vi "Get FIFO Offsets by Name and DataType.vi"(6 "offset":i32, 7 "User Specified?":bool, 8 "error in":errorcluster, 9 "HostToTarget FIFOs":string[](array[string]), 10 "TargetToHost FIFOs":string[](array[string]), 11 "bitfile xml in":string) -> (0 "error out":errorcluster, 1 "HostToTarget":T2, 2 "TargetToHost":T2, 4 "offset past EndTag":i32, 5 "All FIFOs":T1[](array[typedef]))   [LabVIEW 2010, in "FPGA Bitfile Utility.lvlib"]
uses:
  <userlib>/_FPGA Interface Advanced Tools/FPGA Bitfile Utility/FPGA Bitfile Utility.lvlib
  <userlib>/_FPGA Interface Advanced Tools/FPGA Bitfile Utility/TypeDefs/FIFO Channel Set.ctl
  <userlib>/_FPGA Interface Advanced Tools/FPGA Bitfile Utility/TypeDefs/FIFO Channel.ctl
  <vilib>/rvi/DataTransferAndStorage/Container/Common/niFpgaDataTypeControl.ctl
  <userlib>/_FPGA Interface Advanced Tools/FPGA Bitfile Utility/Get FIFOs.vi
  <vilib>/rvi/Utilities/XML/nirviXML_GetValue.vi
  <vilib>/rvi/Utilities/XML/nirviXML_GetValue_String.vi
  resource/RVI/compilationResultUtilities/niLvFpgaGetDmaChannelInfoFromXML.vi
  <vilib>/Utility/error.llb/Error Cluster From Error Code.vi
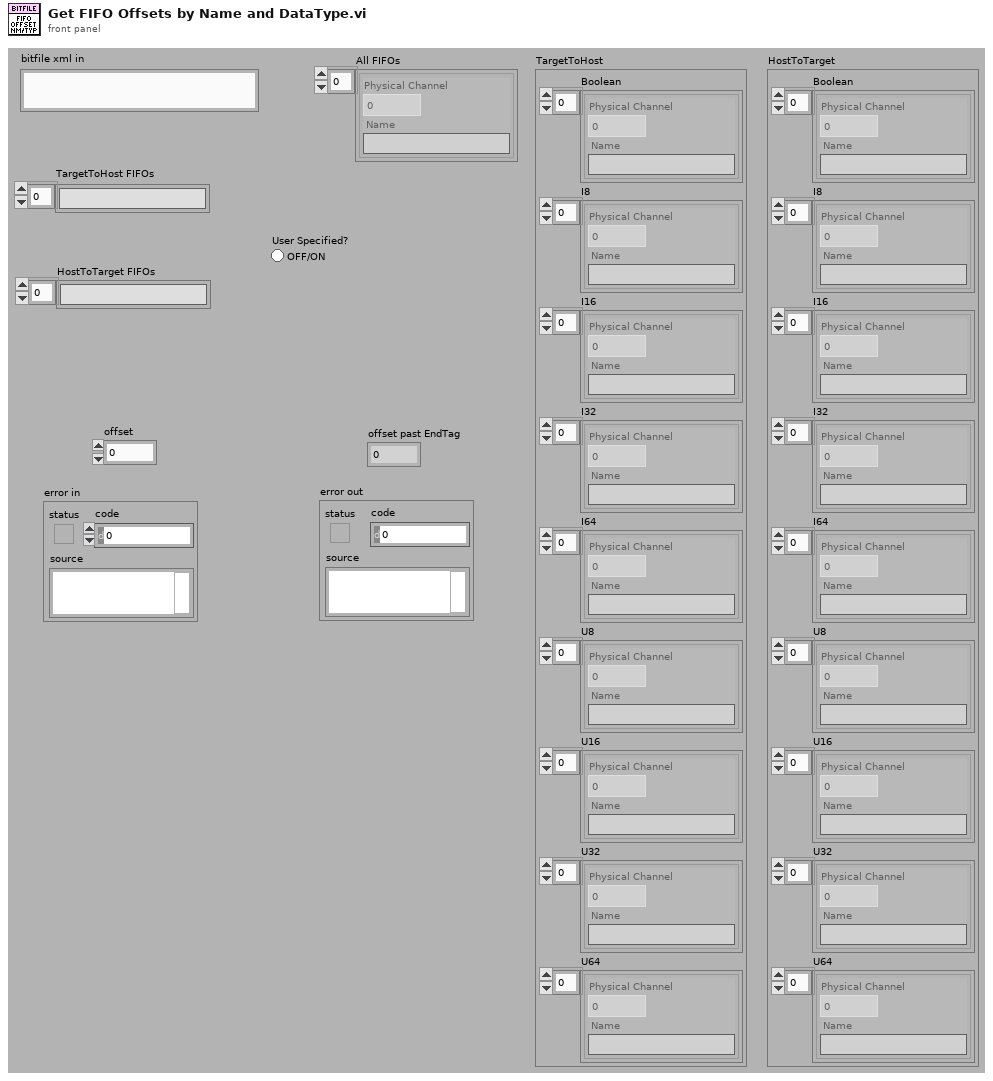
[diagram p1: front panel]
types:
  T1 = typedef "FPGA Bitfile Utility.lvlib/FIFO Channel.ctl" = cluster{"Physical Channel":u32, "Name":string}
  T2 = typedef "FPGA Bitfile Utility.lvlib/FIFO Channel Set.ctl" = cluster{"Boolean":T1[], "I8":T1[], "I16":T1[], "I32":T1[], "I64":T1[], "U8":T1[], "U16":T1[], "U32":T1[], "U64":T1[]}
  T3 = typedef "FPGA Bitfile Utility.lvlib/FIFO Info.ctl" = cluster{"Data Type":T4, "Physical Channel":u32, "Name":string}
  T4 = typedef "niFpgaDataTypeControl.ctl" = enum32{"Boolean", "I8", "I16", "I32", "I64", "U8", "U16", "U32", "U64", "FXP", "CustomControl"}
  T5 = cluster{T1[], T1[], T1[], T1[], T1[], T1[], T1[], T1[], T1[]}
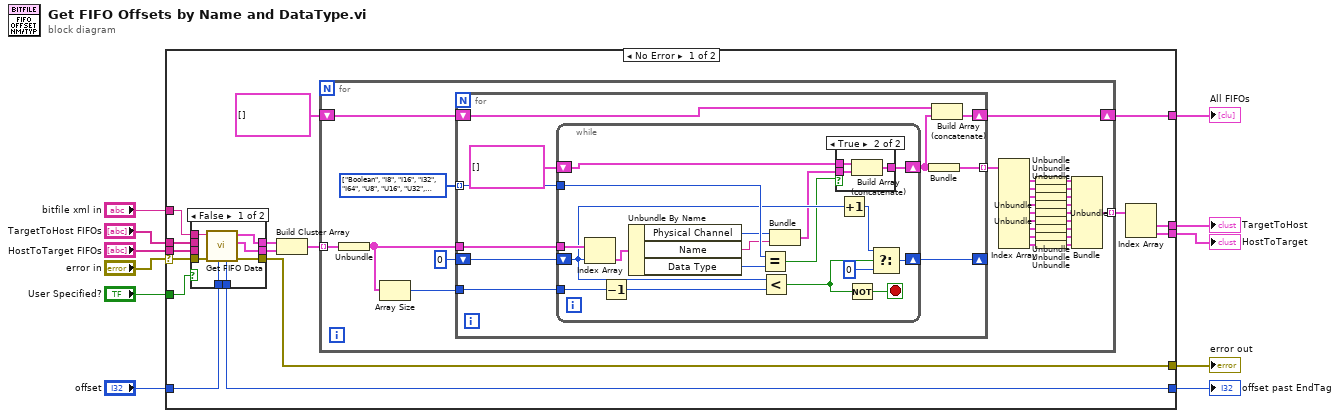
[diagram p0: block diagram]
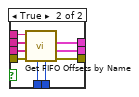
[diagram p2: hidden frame]
diagram:
  n1 = case shown="No Error" "error in" {
    selector: "error in" -> [w20 w104]
    tunnel: [w25 _] -> w4
    tunnel: [w24 _] -> w3
    tunnel: [w21 w104] -> w10
    tunnel: "bitfile xml in" -> [w15 _]
    tunnel: "TargetToHost FIFOs" -> [w19 _]
    tunnel: "HostToTarget FIFOs" -> [w18 _]
    tunnel: "offset" -> [w17 w103]
    tunnel: [w16 w103] -> w5
    tunnel: [w13 _] -> w2
    tunnel: "User Specified?" -> [w12 _]
    frame No Error {
      n2 = case shown="False" w12 {
        tunnel: [w30 w43] -> w23
        tunnel: [w29 w42] -> w22
        tunnel: [w28 w41] -> w21
        tunnel: w20 -> [w31 w40]
        tunnel: w19 -> [_ w39]
        tunnel: w18 -> [_ w38]
        tunnel: w17 -> [w33 w37]
        tunnel: [w32 w36] -> w16
        tunnel: w15 -> [w34 w35]
        frame False {
          n3 = call <userlib>:"Get FIFO Data.vi"("offset"=w33, "error in (no error)"=w31, "bitfile xml in"=w34) -> ("error out"=w28:errorcluster, "HostToTargetFIFOs"=w29:T3[], "TargetToHost FIFOs"=w30:T3[], "offset past EndTag"=w32:i32)  [unwired: 5 in]
        }
        frame True {
          n4 = call <userlib>:"Get FIFO Offsets by Name.vi"("offset"=w37, "error in (no error)"=w40, "HostToTarget FIFOs"=w38, "TargetToHost FIFOs"=w39, "bitfile xml in"=w35) -> ("error out"=w41:errorcluster, "HostToTarget FIFO Offsets"=w42:T3[], "TargetToHost FIFO Offsets"=w43:T3[], "offset past EndTag"=w36:i32)  [unwired: 3 in]
        }
      }
      n5 = Build Cluster Array(w23, w22) -> (w27:cluster{"HostToTarget FIFO Offsets":T3[]}[])
      n6 = for {
        tunnel: w27 -> [w70] mode=indexing
        tunnel: [w46] -> w26 mode=indexing
        shift-right: [w45] -> w13
        shift-left: T1[] [] -> [w44]
        w69 = T4[] [enum."Boolean", enum."I8", enum."I16", enum."I32", enum."I64", enum."U8", enum."U16", enum."U32", enum."U64"] items=["Boolean", "I8", "I16", "I32", "I64", "U8", "U16", "U32", "U64", "FXP", "CustomControl"]
        n7 = Unbundle(w70) -> ("HostToTarget FIFO Offsets"=w66:T3[])
        n8 = Array Size(array=w66) -> (size(s)=w67:i32)
        n9 = for {
          tunnel: w69 -> [w80] mode=indexing
          tunnel: w66 -> [w79]
          shift-right: [w77] -> _
          shift-left: 0 -> [w78]
          tunnel: [w76] -> w47 mode=indexing
          tunnel: w67 -> [w74]
          shift-right: [w72] -> w45
          shift-left: w44 -> [w71]
          n10 = while {
            tunnel: w80 -> [w94]
            tunnel: w79 -> [w98]
            shift-right: [w96] -> w77
            shift-left: w78 -> [w88]
            shift-right: [w92] -> w73
            shift-left: T1[] [] -> [w91]
            tunnel: w74 -> [w89]
            stop <- w90 stop-if-true
            n11 = Index Array(array=w98, index=w88) -> (element=w93:T3)
            n12 = Decrement(x=w89) -> (x-1=w84:i32)
            n13 = Unbundle By Name(w93) -> ("Physical Channel"=w87:u32, "Name"=w86:string, "Data Type"=w95:T4)
            n14 = Equal?(x=w94, y=w95) -> (x = y?=w82:bool)
            n15 = Less?(x=w88, y=w84) -> (x < y?=w83:bool)
            n16 = Bundle("Physical Channel"=w87, "Name"=w86) -> (w85:cluster{"Physical Channel":u32, "Name":string})  [unwired: 1 in]
            n17 = case shown="True" w82 {
              tunnel: w85 -> [_ w102]
              tunnel: [w99 w101] -> w92
              tunnel: w91 -> [w99 w100]
              frame False {
              }
              frame True {
                n18 = Build Array (concatenate)(w100, w102) -> (w101:T1[])
              }
            }
            n19 = Increment(x=w88) -> (x+1=w97:i32)
            n20 = Not(x=w83) -> (.not. x?=w90:bool)
            n21 = Select(t=w97, s=w83, f=0) -> (s? t:f=w96:i32)
          }
          n22 = Bundle(w73) -> (w76:cluster{T1[]})  [unwired: 1 in]
          n23 = Build Array (concatenate)(w71, w73) -> (w72:T1[])
        }
        n24 = Index Array(array=w47) -> (element #1=w48:cluster{T1[]}, element #2=w50:cluster{T1[]}, element #3=w52:cluster{T1[]}, element #4=w53:cluster{T1[]}, element #5=w56:cluster{T1[]}, element #6=w57:cluster{T1[]}, element #7=w58:cluster{T1[]}, element #8=w59:cluster{T1[]}, element #9=w60:cluster{T1[]})  [unwired: 9 in]
        n25 = Unbundle(w48) -> (w49:T1[])
        n26 = Unbundle(w50) -> (w51:T1[])
        n27 = Unbundle(w52) -> (w55:T1[])
        n28 = Unbundle(w53) -> (w54:T1[])
        n29 = Unbundle(w56) -> (w65:T1[])
        n30 = Unbundle(w57) -> (w64:T1[])
        n31 = Unbundle(w58) -> (w63:T1[])
        n32 = Unbundle(w59) -> (w62:T1[])
        n33 = Unbundle(w60) -> (w61:T1[])
        n34 = Bundle(w49, w51, w55, w54, w65, w64, w63, w62, w61) -> (w46:T5)  [unwired: 1 in]
      }
      n35 = Index Array(array=w26) -> (element #1=w25:T5, element #2=w24:T5)  [unwired: 2 in]
    }
    frame Error {
    }
  }
  "error out" <- w10
  "offset past EndTag" <- w5
  "TargetToHost" <- w4
  "HostToTarget" <- w3
  "All FIFOs" <- w2
